vi "Inst_CNT90.vi"(8 "error in":errorcluster, 10 "All Message Queues in":T1, 11 "Prueba31 in":refnum<class "Prueba10.lvclass">) -> (0 "error out":errorcluster)   [LabVIEW 2019, in "Prueba10.lvclass"]
uses:
  Prueba10.lvclass
  QMH/Message Queue/All Message Queues.ctl
  QMH/Message Queue/Message Cluster.ctl
  Prueba10.lvclass/Prueba10.ctl
  <vilib>/Utility/error.llb/Error Cluster From Error Code.vi
  QMH/Message Queue/Enqueue Message (Single).vi
  <vilib>/ErrorRing/Error Ring.xnode
  QMH/Message Queue/Message Queue.lvlib
  Instrumento/CNT90/CNT90.lvclass
panel:
  out "All States":string[](array[string])
  out "Actual State":string
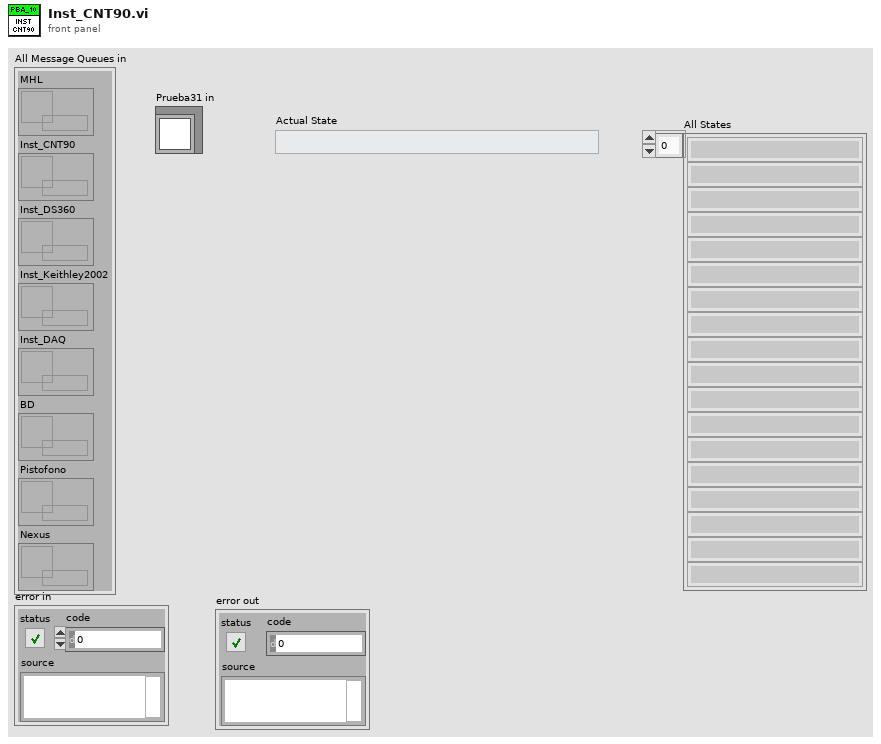
[diagram p1: front panel]
types:
  T1 = typedef "Message Queue.lvlib/All Message Queues.ctl" = cluster{"MHL":refnum<queue>, "Inst_CNT90":refnum<queue>, "Inst_DS360":refnum<queue>, "Inst_Keithley2002":refnum<queue>, "Inst_DAQ":refnum<queue>, "BD":refnum<queue>, "Pistofono":refnum<queue>, "Nexus":refnum<queue>}
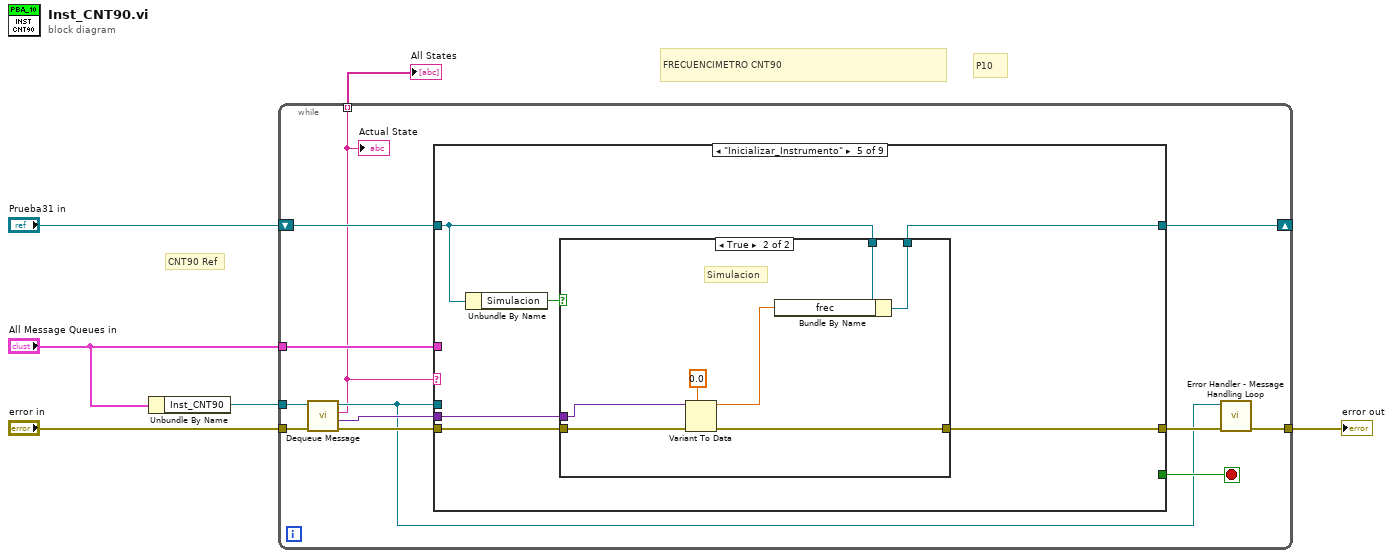
[diagram p0: block diagram]
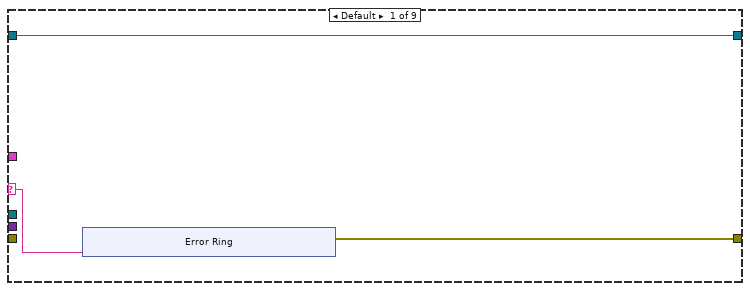
[diagram p2: hidden frame]
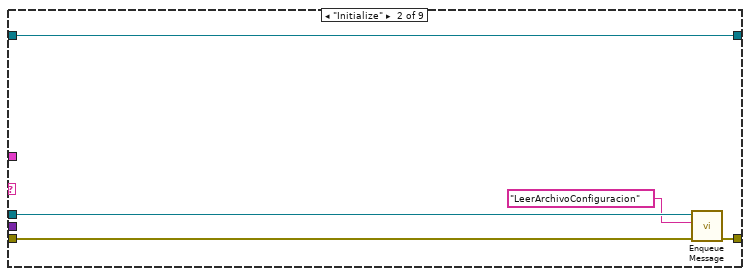
[diagram p3: hidden frame]
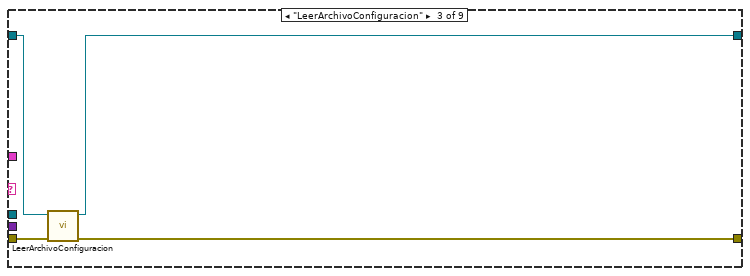
[diagram p4: hidden frame]
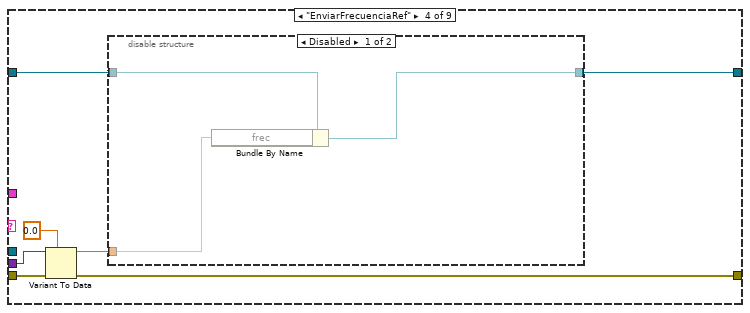
[diagram p5: hidden frame]
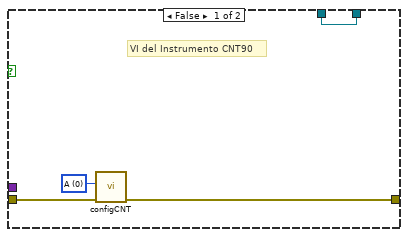
[diagram p7: hidden frame]
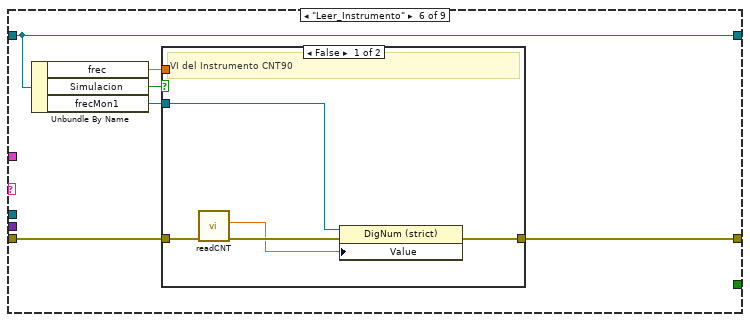
[diagram p8: hidden frame]
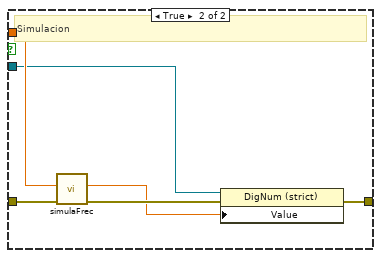
[diagram p9: hidden frame]
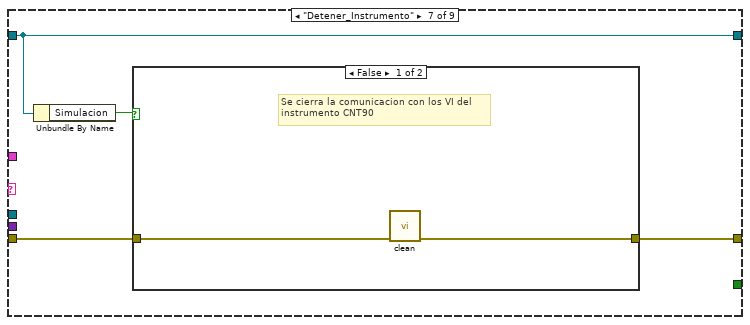
[diagram p10: hidden frame]
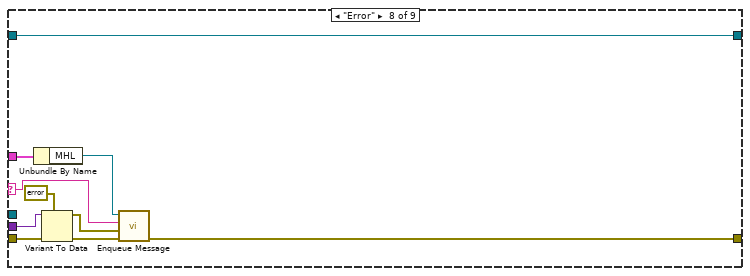
[diagram p12: hidden frame]
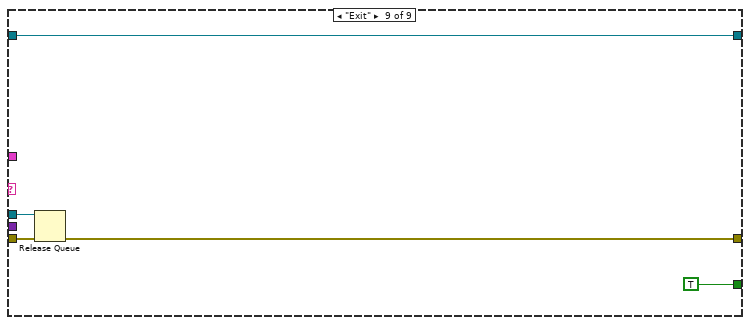
[diagram p13: hidden frame]
diagram:
  # "P10"
  # "FRECUENCIMETRO CNT90"
  # "CNT90 Ref"
  n1 = Unbundle By Name("All Message Queues in") -> ("Inst_CNT90"=w4:refnum<queue>)
  n2 = while {
    tunnel: "error in" -> [w18]
    tunnel: w4 -> [w17]
    tunnel: "All Message Queues in" -> [w16]
    tunnel: [w9] -> w2
    shift-right: [w12] -> _
    shift-left: "Prueba31 in" -> [w15]
    tunnel: [w7] -> w1 mode=indexing
    stop <- w11 stop-if-true
    n3 = call "Dequeue Message.vi"("error in (no error)"=w18, "Message Queue"=w17) -> ("error out"=w13:errorcluster, "Message Data"=w14:variant, "Message"=w7:string, "dup Message Queue"=w8:refnum<queue>)  [unwired: 6 in]
    "Actual State" <- w7
    n4 = case shown="\"Inicializar_Instrumento\"" w7 {
      selector: w7 -> [w21 _ _ _ _ _ _ w94 _]
      tunnel: w16 -> [_ _ _ _ _ _ _ w93 _]
      tunnel: w15 -> [w19 w33 w34 w39 w50 w69 w85 w91 w101]
      tunnel: w8 -> [_ w30 _ _ _ _ _ _ w103]
      tunnel: w14 -> [_ _ _ w42 w51 _ _ w97 _]
      tunnel: w13 -> [_ w31 w35 w43 w54 w71 w83 w98 w104]
      tunnel: [w20 w32 w37 w44 w52 w70 w86 w90 w100] -> w10
      tunnel: [w19 w33 w36 w40 w49 w69 w85 w91 w101] -> w12
      tunnel: [_ _ _ _ _ _ _ _ TRUE] -> w11
      frame Default {
        n5 = xnode "Error Ring"("parameter 0"=w21) -> ("error out"=w20:errorcluster)
      }
      frame "Initialize" {
        n6 = call-poly "Enqueue Message.vi"("error in (no error)"=w31, "Message"="LeerArchivoConfiguracion", "Message Queue"=w30) -> ("error out"=w32:errorcluster)  [unwired: 7 in, 1 out]
      }
      frame "LeerArchivoConfiguracion" {
        n7 = call "LeerArchivoConfiguracion.vi"("error in"=w35, "Prueba10 in"=w34) -> ("error out"=w37:errorcluster, "Prueba10 out"=w36:refnum<class "Prueba10.lvclass">)  [unwired: 8 in]
      }
      frame "EnviarFrecuenciaRef" {
        n8 = Variant To Data(error in=w43, type=0.0, Variant=w42) -> (data=w38:dbl, error out=w44:errorcluster)
        n9 = disable-structure shown="Disabled" {
          disable-tunnel: [w47 w48] -> w40
          disable-tunnel: w39 -> [w46 w48]
          disable-tunnel: w38 -> [w45 _]
          frame Disabled {
            n10 = Bundle By Name(cluster=w46, "frec"=w45) -> (w47:refnum<class "Prueba10.lvclass">)
          }
          frame Enabled {
          }
        }
      }
      frame "Inicializar_Instrumento" {
        n11 = Unbundle By Name(w50) -> ("Simulacion"=w53:bool)
        n12 = case shown="True" w53 {
          tunnel: [w58 w64] -> w52
          tunnel: w54 -> [w57 w65]
          tunnel: w51 -> [_ w63]
          tunnel: w50 -> [w55 w62]
          tunnel: [w55 w61] -> w49
          frame False {
            w56 = 0 items=["A", "B"] ("Channel  1")
            # "VI del Instrumento CNT90"
            n13 = call "configCNT.vi"("error in (no error)"=w57, "Channel  1"=w56) -> ("error out"=w58:errorcluster)  [unwired: 8 in, 1 out]
          }
          frame True {
            # "Simulacion"
            n14 = Variant To Data(error in=w65, type=0.0 ("frecuencia"), Variant=w63) -> (data=w60:dbl, error out=w64:errorcluster)
            n15 = Bundle By Name(cluster=w62, "frec"=w60) -> (w61:refnum<class "Prueba10.lvclass">)
          }
        }
      }
      frame "Leer_Instrumento" {
        n16 = Unbundle By Name(w69) -> ("frec"=w67:dbl, "Simulacion"=w68:bool, "frecMon1"=w66:refnum<vi>)
        n17 = case shown="False" w68 {
          tunnel: [w74 w79] -> w70
          tunnel: w71 -> [w76 w82]
          tunnel: w67 -> [_ w81]
          tunnel: w66 -> [w73 w78]
          frame False {
            # "VI del Instrumento CNT90"
            n18 = call "readCNT.vi"("error in (no error)"=w76) -> ("error out"=w75:errorcluster, "medicion"=w72:dbl)  [unwired: 8 in, 1 out]
            n19 = property class="DigNum (strict)"(reference=w73, error in=w75, "Value"=w72) -> (error out=w74:errorcluster)  [unwired: 1 out]
          }
          frame True {
            # "Simulacion"
            n20 = call "simulaFrec.vi"("error in (no error)"=w82, "frec in"=w81) -> ("error out"=w80:errorcluster, "frec out"=w77:dbl)  [unwired: 7 in, 1 out]
            n21 = property class="DigNum (strict)"(reference=w78, error in=w80, "Value"=w77) -> (error out=w79:errorcluster)  [unwired: 1 out]
          }
        }
      }
      frame "Detener_Instrumento" {
        n22 = Unbundle By Name(w85) -> ("Simulacion"=w84:bool)
        n23 = case shown="False" w84 {
          tunnel: [w88 w89] -> w86
          tunnel: w83 -> [w87 w89]
          frame False {
            # "Se cierra la comunicacion con los VI del\ninstrumento CNT90"
            n24 = call "clean.vi"("error in (no error)"=w87) -> ("error out"=w88:errorcluster)  [unwired: 9 in, 1 out]
          }
          frame True {
            # "Simulacion"
          }
        }
      }
      frame "Error" {
        n25 = Unbundle By Name(w93) -> ("MHL"=w92:refnum<queue>)
        n26 = Variant To Data(error in=w98, type=errorcluster {"status"=FALSE, "code"=0, "source"=""} ("error constant"), Variant=w97) -> (data=w95:errorcluster, error out=w96:errorcluster)
        n27 = call-poly "Enqueue Message.vi"("error in (no error)"=w96, "Message Data"=w95, "Message"=w94, "Message Queue"=w92) -> ("error out"=w90:errorcluster)  [unwired: 6 in, 1 out]
      }
      frame "Exit" {
        n28 = Release Queue(queue=w103, error in (no error)=w104) -> (error out=w100:errorcluster)  [unwired: 1 in, 2 out]
      }
    }
    n29 = call "Error Handler - Message Handling Loop.vi"("error in (no error)"=w10, "Message Queue"=w8) -> ("dup error in"=w9:errorcluster)  [unwired: 8 in, 1 out]
  }
  "error out" <- w2
  "All States" <- w1
